vi "发送数据.vi"(1 "发送数据":string, 2 "VISA资源名称":refnum<visa-resource-name>) -> ()   [LabVIEW 2017]
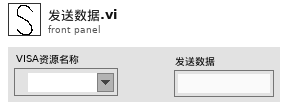
[diagram p1: front panel]
types:
  T1 = enum16{"Native", "Native Command Line", "UNIX", "Macintosh", "DOS"}
  T2 = enum16{"big-endian, network order", "native, host order", "little-endian"}
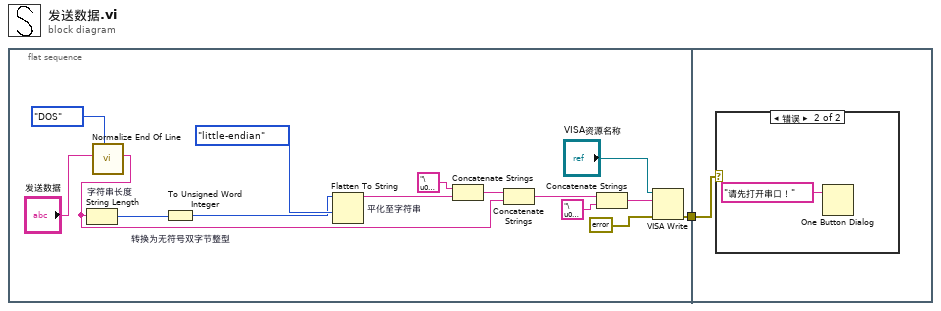
[diagram p0: block diagram]
diagram:
  n1 = flat-sequence {
    tunnel: [w2] -> w1
    tunnel: w1 -> [w17]
    frame #0 {
      n2 = call <vilib>:"Normalize End Of Line.vi"("end of line (Native)"=T1."DOS", "string in"="发送数据") -> ("string out"=w4:string)  [unwired: 6 in]
      n3 = String Length "字符串长度"(string=w4) -> (length=w15:i32)
      n4 = To Unsigned Word Integer "转换为无符号双字节整型"(number=w15) -> (unsigned 16bit integer=w7:u16)
      n5 = Flatten To String "平化至字符串"(anything=w7, byte order (0:big-endian, network order)=T2."little-endian" ("字节顺序(0:big-endian, network order)")) -> (data string=w14:string)  [unwired: 2 in, 2 out]
      n6 = Concatenate Strings("\u0002" ("字符串"), w14) -> (w13:string)
      n7 = Concatenate Strings(w13, w4) -> (w12:string)
      n8 = Concatenate Strings(w12, "\u0003" ("字符串")) -> (w9:string)
      n9 = VISA Write(VISA resource name="VISA资源名称", write buffer=w9, error in (no error)=errorcluster {"status"=FALSE, "code"=0, "source"=""} ("错误输入（无错误）")) -> (error out=w2:errorcluster)  [unwired: 2 out]
    }
    frame #1 {
      n10 = case shown="错误" w17 {
        frame No Error {
        }
        frame Error {
          n11 = One Button Dialog(message="请先打开串口！" ("消息")) -> ()  [unwired: 1 in, 1 out]
        }
      }
    }
  }
